vi "PrefDialog_Tabs.vi"(8 "error in (no error)":errorcluster, 11 "MyPluginsBase in":refnum<class "NHRGridSim.lvclass">) -> (0 "error out":errorcluster, 1 "Save As":bool, 2 "Changed":bool, 3 "MyPluginsBase out":refnum<class "NHRGridSim.lvclass">)   [LabVIEW 2018, in "AcPwrPlugins.lvlib" / "NHRGridSim.lvclass"]
doc: "This VI opens up the modal preference dialog window and allows a user to configure the properties with new values, or keep the existing values from the last time the function was called. The user can also save the new values to a new file name and new type name using the save as button."
uses:
  NHRGridSim.lvclass
  TypeDefs/NHRGrid_InstrumentCluster_Tabs.ctl
  TypeDefs/NHRGrid_Phases.ctl
  TypeDefs/NHRGrid_SlewRates_Tabs.ctl
  TypeDefs/NHRGrid_Configure_Tabs.ctl
  TypeDefs/NHRGrid_WaveShape_Tabs.ctl
  TypeDefs/NHRGrid_Ranges_Tabs.ctl
  TypeDefs/NHRGrid_SafetyTrips_Tabs.ctl
  Measurements.ctl
  TypeDefs/MeasurementType.ctl
  TypeDefs/NHRGrid_Modes.ctl
  TypeDefs/NHRGrid_ModeAdjust_Tabs.ctl
  <vilib>/Utility/config.llb/NI_LVConfig.lvlib
  AcPwrBaseClass/AcPwrBase.lvclass
panel:
  in  "MeasName":string
  in  "Connected":bool
  in  "ID Query":bool
  in  "Mode":T1 items=["3-Phase AC"=0, "AC"=1, "DC"=2, "AC - AC"=7, "AC - DC"=8, "DC - AC"=11, "DC - DC"=12, "2-Phase AC - AC"=5, "2-Phase AC - DC"=6, "AC - AC - AC"=3, "DC - DC - DC"=4, "AC - AC - DC"=9, "AC - DC - DC"=10, "AC - DC - AC"=13, "DC - AC - AC"=14, "DC - AC - DC"=15]
  in  "Reset":bool
  in  "Handle":string
  in  "Instruments":enum32{"Page 1", "Page 2", "Page 3"}(tab)
  in  "Instr1":T2={"Name"="", "Vout (V)"=0.0, "VType"="", "Phases"={"A-Volts (V)"=0.0, "B-Volts (V)"=0.0, "C-Volts (V)"=0.0, "Change at (Deg)"=0.0, "B-Angle (Deg)"=240.0, "C-Angle (Deg)"=120.0}, "Slew Rates"={"Vmax (V/s)"=0.0, "Vmin (V/s)"=0.0, "Imax (A/s)"=0.0, "Imin (A/s)"=0.0, "Pmax (W/s)"=0.0, "Pmin (W/s)"=0.0, "Freq Max (Hz/s)"=0.0, "Freq Min (Hz/s)"=0.0, "Ph Angle Max (Deg/s)"=0.0, "Ph Angle Min (Deg/s)"=0.0}, "FreqOut (Hz)"=60.0, "Aperture (cycles)"=1, "Configure Instrument"=0, "AC Wave Shape"=0, "Ranges"={"Voltage (V)"=0, "Current (A)"=606}, "Safety Trips"={"Vmax (V)"=0.0, "Vmin (V)"=0.0, "Vmax Time (s)"=-1.0, "Vmin Time (s)"=-1.0, "Imax Source (A)"=0.0, "Imax Sink (A)"=0.0, "I Src Time (s)"=-1.0, "I Snk Time (s)"=-1.0, "Pmax Source (W)"=0.0, "Pmax Sink (W)"=0.0, "P Src Time (s)"=-1.0, "P Snk Time (s)"=-1.0, "Abs Volt Peak"=0.0, "Enable Vpk"=FALSE, "Abs Curr Peak"=0.0, "Enable Ipk"=FALSE}} {"Safety Trips"."Abs Curr Peak" min=0.0; "Safety Trips"."Abs Volt Peak" min=0.0; "Safety Trips"."P Snk Time (s)" min=-1.0; "Safety Trips"."Pmax Sink (W)" min=0.0 format="%#_7g"; "Safety Trips"."P Src Time (s)" min=-1.0; "Safety Trips"."Pmax Source (W)" min=0.0 format="%#_7g"; "Safety Trips"."I Snk Time (s)" min=-1.0; "Safety Trips"."Imax Sink (A)" min=0.0; "Safety Trips"."I Src Time (s)" min=-1.0; "Safety Trips"."Imax Source (A)" min=0.0; "Safety Trips"."Vmax Time (s)" min=-1.0; "Safety Trips"."Vmax (V)" min=0.0; "Safety Trips"."Vmin Time (s)" min=-1.0; "Safety Trips"."Vmin (V)" min=0.0; "Ranges"."Current (A)" items=["200", "400"]; "Ranges"."Voltage (V)" items=["200", "400"]; "AC Wave Shape" items=["Sine", "User1", "User2", "User3"]; "Configure Instrument" items=["Immediate", "Sync to Phase A"]; "Aperture (cycles)" min=1 max=64; "FreqOut (Hz)" min=0.0 max=100.0; "Slew Rates"."Ph Angle Min (Deg/s)" min=0.0; "Slew Rates"."Ph Angle Max (Deg/s)" min=0.0; "Slew Rates"."Freq Min (Hz/s)" min=0.0; "Slew Rates"."Freq Max (Hz/s)" min=0.0; "Slew Rates"."Pmax (W/s)" min=0.0; "Slew Rates"."Pmin (W/s)" min=0.0; "Slew Rates"."Imax (A/s)" min=0.0; "Slew Rates"."Vmax (V/s)" min=0.0; "Slew Rates"."Imin (A/s)" min=0.0; "Slew Rates"."Vmin (V/s)" min=0.0; "Phases"."Change at (Deg)" min=0.0; "Phases"."C-Angle (Deg)" min=0.0; "Phases"."B-Angle (Deg)" min=0.0; "Phases"."C-Volts (V)" min=0.0; "Phases"."B-Volts (V)" min=0.0; "Phases"."A-Volts (V)" min=0.0; "Vout (V)" min=0.0}
  in  "Instr2":T2={"Name"="", "Vout (V)"=0.0, "VType"="", "Phases"={"A-Volts (V)"=0.0, "B-Volts (V)"=0.0, "C-Volts (V)"=0.0, "Change at (Deg)"=0.0, "B-Angle (Deg)"=240.0, "C-Angle (Deg)"=120.0}, "Slew Rates"={"Vmax (V/s)"=0.0, "Vmin (V/s)"=0.0, "Imax (A/s)"=0.0, "Imin (A/s)"=0.0, "Pmax (W/s)"=0.0, "Pmin (W/s)"=0.0, "Freq Max (Hz/s)"=0.0, "Freq Min (Hz/s)"=0.0, "Ph Angle Max (Deg/s)"=0.0, "Ph Angle Min (Deg/s)"=0.0}, "FreqOut (Hz)"=60.0, "Aperture (cycles)"=1, "Configure Instrument"=0, "AC Wave Shape"=0, "Ranges"={"Voltage (V)"=0, "Current (A)"=606}, "Safety Trips"={"Vmax (V)"=0.0, "Vmin (V)"=0.0, "Vmax Time (s)"=-1.0, "Vmin Time (s)"=-1.0, "Imax Source (A)"=0.0, "Imax Sink (A)"=0.0, "I Src Time (s)"=-1.0, "I Snk Time (s)"=-1.0, "Pmax Source (W)"=0.0, "Pmax Sink (W)"=0.0, "P Src Time (s)"=-1.0, "P Snk Time (s)"=-1.0, "Abs Volt Peak"=0.0, "Enable Vpk"=FALSE, "Abs Curr Peak"=0.0, "Enable Ipk"=FALSE}} {"Safety Trips"."Abs Curr Peak" min=0.0; "Safety Trips"."Abs Volt Peak" min=0.0; "Safety Trips"."P Snk Time (s)" min=-1.0; "Safety Trips"."Pmax Sink (W)" min=0.0 format="%#_7g"; "Safety Trips"."P Src Time (s)" min=-1.0; "Safety Trips"."Pmax Source (W)" min=0.0 format="%#_7g"; "Safety Trips"."I Snk Time (s)" min=-1.0; "Safety Trips"."Imax Sink (A)" min=0.0; "Safety Trips"."I Src Time (s)" min=-1.0; "Safety Trips"."Imax Source (A)" min=0.0; "Safety Trips"."Vmax Time (s)" min=-1.0; "Safety Trips"."Vmax (V)" min=0.0; "Safety Trips"."Vmin Time (s)" min=-1.0; "Safety Trips"."Vmin (V)" min=0.0; "Ranges"."Current (A)" items=["6", "30"]; "Ranges"."Voltage (V)" items=["175", "350"]; "AC Wave Shape" items=["Sine", "User1", "User2", "User3"]; "Configure Instrument" items=["Immediate", "Sync to Phase A"]; "Aperture (cycles)" min=1 max=64; "FreqOut (Hz)" min=0.0 max=100.0; "Slew Rates"."Ph Angle Min (Deg/s)" min=0.0; "Slew Rates"."Ph Angle Max (Deg/s)" min=0.0; "Slew Rates"."Freq Min (Hz/s)" min=0.0; "Slew Rates"."Freq Max (Hz/s)" min=0.0; "Slew Rates"."Pmax (W/s)" min=0.0; "Slew Rates"."Pmin (W/s)" min=0.0; "Slew Rates"."Imax (A/s)" min=0.0; "Slew Rates"."Vmax (V/s)" min=0.0; "Slew Rates"."Imin (A/s)" min=0.0; "Slew Rates"."Vmin (V/s)" min=0.0; "Phases"."Change at (Deg)" min=0.0; "Phases"."C-Angle (Deg)" min=0.0; "Phases"."B-Angle (Deg)" min=0.0; "Phases"."C-Volts (V)" min=0.0; "Phases"."B-Volts (V)" min=0.0; "Phases"."A-Volts (V)" min=0.0; "Vout (V)" min=0.0}
  in  "Instr3":T2={"Name"="", "Vout (V)"=0.0, "VType"="", "Phases"={"A-Volts (V)"=0.0, "B-Volts (V)"=0.0, "C-Volts (V)"=0.0, "Change at (Deg)"=0.0, "B-Angle (Deg)"=240.0, "C-Angle (Deg)"=120.0}, "Slew Rates"={"Vmax (V/s)"=0.0, "Vmin (V/s)"=0.0, "Imax (A/s)"=0.0, "Imin (A/s)"=0.0, "Pmax (W/s)"=0.0, "Pmin (W/s)"=0.0, "Freq Max (Hz/s)"=0.0, "Freq Min (Hz/s)"=0.0, "Ph Angle Max (Deg/s)"=0.0, "Ph Angle Min (Deg/s)"=0.0}, "FreqOut (Hz)"=60.0, "Aperture (cycles)"=1, "Configure Instrument"=0, "AC Wave Shape"=0, "Ranges"={"Voltage (V)"=0, "Current (A)"=606}, "Safety Trips"={"Vmax (V)"=0.0, "Vmin (V)"=0.0, "Vmax Time (s)"=-1.0, "Vmin Time (s)"=-1.0, "Imax Source (A)"=0.0, "Imax Sink (A)"=0.0, "I Src Time (s)"=-1.0, "I Snk Time (s)"=-1.0, "Pmax Source (W)"=0.0, "Pmax Sink (W)"=0.0, "P Src Time (s)"=-1.0, "P Snk Time (s)"=-1.0, "Abs Volt Peak"=0.0, "Enable Vpk"=FALSE, "Abs Curr Peak"=0.0, "Enable Ipk"=FALSE}} {"Safety Trips"."Abs Curr Peak" min=0.0; "Safety Trips"."Abs Volt Peak" min=0.0; "Safety Trips"."P Snk Time (s)" min=-1.0; "Safety Trips"."Pmax Sink (W)" min=0.0 format="%#_7g"; "Safety Trips"."P Src Time (s)" min=-1.0; "Safety Trips"."Pmax Source (W)" min=0.0 format="%#_7g"; "Safety Trips"."I Snk Time (s)" min=-1.0; "Safety Trips"."Imax Sink (A)" min=0.0; "Safety Trips"."I Src Time (s)" min=-1.0; "Safety Trips"."Imax Source (A)" min=0.0; "Safety Trips"."Vmax Time (s)" min=-1.0; "Safety Trips"."Vmax (V)" min=0.0; "Safety Trips"."Vmin Time (s)" min=-1.0; "Safety Trips"."Vmin (V)" min=0.0; "Ranges"."Current (A)" items=["6", "30"]; "Ranges"."Voltage (V)" items=["200", "400"]; "AC Wave Shape" items=["Sine", "User1", "User2", "User3"]; "Configure Instrument" items=["Immediate", "Sync to Phase A"]; "Aperture (cycles)" min=1 max=64; "FreqOut (Hz)" min=0.0 max=100.0; "Slew Rates"."Ph Angle Min (Deg/s)" min=0.0; "Slew Rates"."Ph Angle Max (Deg/s)" min=0.0; "Slew Rates"."Freq Min (Hz/s)" min=0.0; "Slew Rates"."Freq Max (Hz/s)" min=0.0; "Slew Rates"."Pmax (W/s)" min=0.0; "Slew Rates"."Pmin (W/s)" min=0.0; "Slew Rates"."Imax (A/s)" min=0.0; "Slew Rates"."Vmax (V/s)" min=0.0; "Slew Rates"."Imin (A/s)" min=0.0; "Slew Rates"."Vmin (V/s)" min=0.0; "Phases"."Change at (Deg)" min=0.0; "Phases"."C-Angle (Deg)" min=0.0; "Phases"."B-Angle (Deg)" min=0.0; "Phases"."C-Volts (V)" min=0.0; "Phases"."B-Volts (V)" min=0.0; "Phases"."A-Volts (V)" min=0.0; "Vout (V)" min=0.0}
  in  "Measurements":T9 {"Instrument Number" items=["1", "2", "3"]}
  in  "btnSaveAs":bool
  in  "Measurement RefreshTime (ms)":u32
  in  "btnSave":bool
  in  "btnCancel":bool
  # "Voltages (L-N)"
  # "Voltages (L-N)"
  # "Voltages (L-N)"
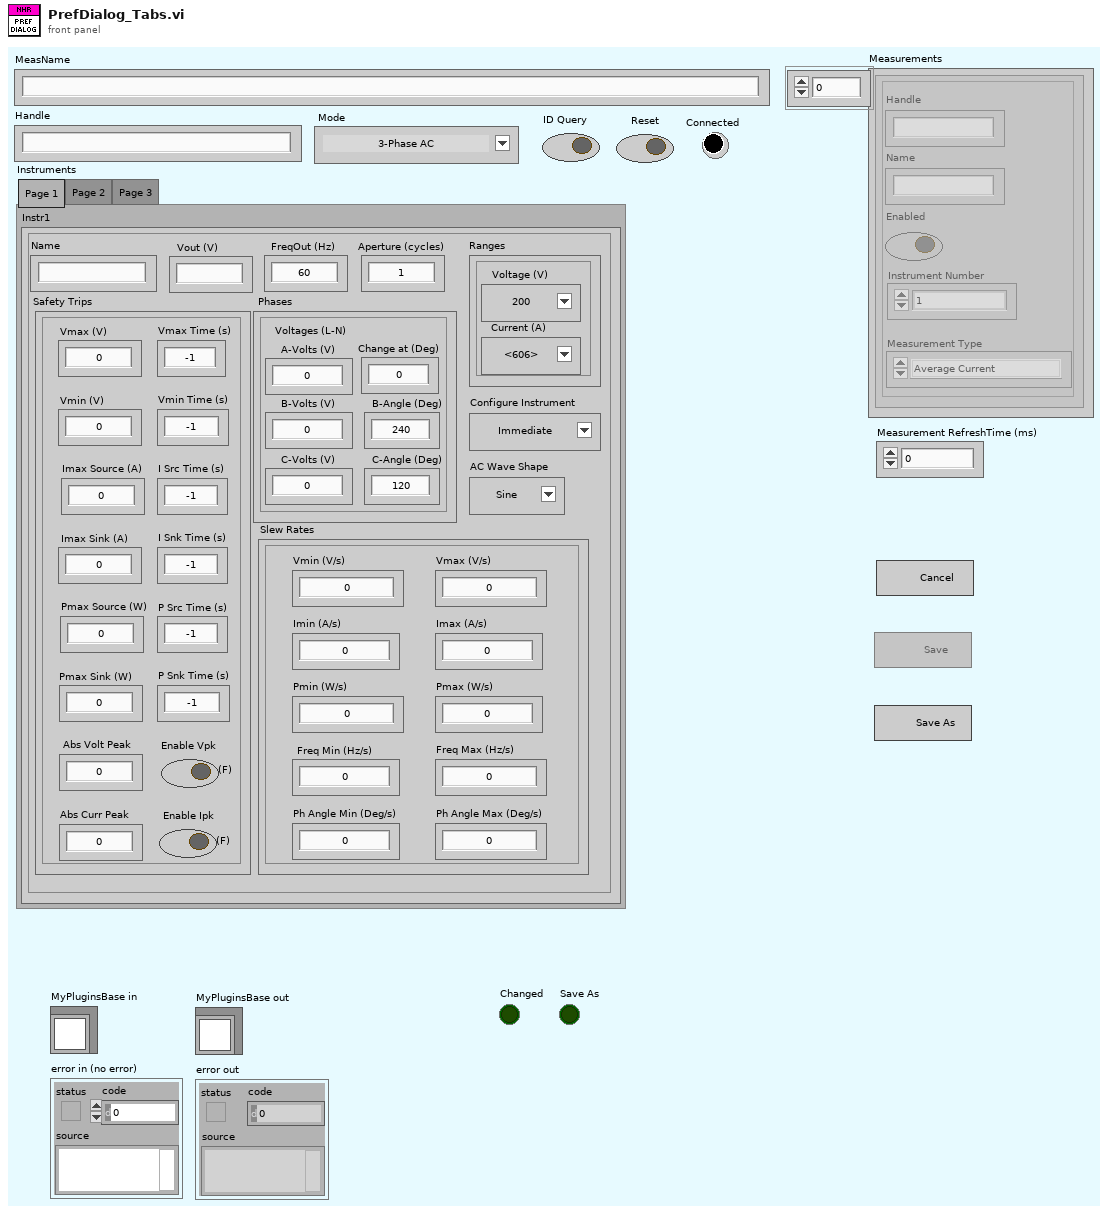
[diagram p1: front panel]
types:
  T1 = typedef "AcPwrPlugins.lvlib/NHRGridSim.lvclass/NHRGrid_Modes.ctl" = u8
  T2 = typedef "AcPwrPlugins.lvlib/NHRGridSim.lvclass/NHRGrid_InstrumentCluster_Tabs.ctl" = cluster{"Name":string, "Vout (V)":dbl, "VType":string, "Phases":T3, "Slew Rates":T4, "FreqOut (Hz)":dbl, "Aperture (cycles)":i32, "Configure Instrument":T5, "AC Wave Shape":T6, "Ranges":T7, "Safety Trips":T8}
  T3 = typedef "AcPwrPlugins.lvlib/NHRGridSim.lvclass/NHRGrid_Phases.ctl" = cluster{"A-Volts (V)":dbl, "B-Volts (V)":dbl, "C-Volts (V)":dbl, "Change at (Deg)":dbl, "B-Angle (Deg)":dbl, "C-Angle (Deg)":dbl}
  T4 = typedef "AcPwrPlugins.lvlib/NHRGridSim.lvclass/NHRGrid_SlewRates_Tabs.ctl" = cluster{"Vmax (V/s)":dbl, "Vmin (V/s)":dbl, "Imax (A/s)":dbl, "Imin (A/s)":dbl, "Pmax (W/s)":dbl, "Pmin (W/s)":dbl, "Freq Max (Hz/s)":dbl, "Freq Min (Hz/s)":dbl, "Ph Angle Max (Deg/s)":dbl, "Ph Angle Min (Deg/s)":dbl}
  T5 = typedef "AcPwrPlugins.lvlib/NHRGridSim.lvclass/NHRGrid_Configure_Tabs.ctl" = u16
  T6 = typedef "AcPwrPlugins.lvlib/NHRGridSim.lvclass/NHRGrid_WaveShape_Tabs.ctl" = u16
  T7 = typedef "AcPwrPlugins.lvlib/NHRGridSim.lvclass/NHRGrid_Ranges_Tabs.ctl" = cluster{"Voltage (V)":u16, "Current (A)":u16}
  T8 = typedef "AcPwrPlugins.lvlib/NHRGridSim.lvclass/NHRGrid_SafetyTrips_Tabs.ctl" = cluster{"Vmax (V)":dbl, "Vmin (V)":dbl, "Vmax Time (s)":dbl, "Vmin Time (s)":dbl, "Imax Source (A)":dbl, "Imax Sink (A)":dbl, "I Src Time (s)":dbl, "I Snk Time (s)":dbl, "Pmax Source (W)":dbl, "Pmax Sink (W)":dbl, "P Src Time (s)":dbl, "P Snk Time (s)":dbl, "Abs Volt Peak":dbl, "Enable Vpk":bool, "Abs Curr Peak":dbl, "Enable Ipk":bool}
  T9 = typedef "AcPwrPlugins.lvlib/NHRGridSim.lvclass/Measurements.ctl" = cluster{"Handle":string, "Name":string, "Enabled ":bool, "Measurement Value":dbl, "Instrument Number ":i32, "Measurement Type ":T10}[]
  T10 = typedef "AcPwrPlugins.lvlib/NHRGridSim.lvclass/MeasurementType.ctl" = enum16{"Average Current", "Average Voltage"}
  T11 = enum32{"Invalid", "Default", "Floating", "Floating/Auto-Hide", "Modal"}
  T12 = enum32{"Invalid", "Standard", "Closed", "Hidden", "Minimized", "Maximized"}
  T13 = typedef "AcPwrPlugins.lvlib/NHRGridSim.lvclass/NHRGrid_ModeAdjust_Tabs.ctl" = enum16{"ShowTabs", "InstrNames", "VoltRanges", "ConfigOpts"}
  T14 = enum8{"Enabled", "Disabled", "Disabled and Grayed Out"}
  T15 = typedef "AcPwrPlugins.lvlib/AcPwrBase.lvclass/BaseConfig.ctl" = cluster{"Frequency":dbl, "FrequencyRange":dbl[], "Phases":T16[], "Name":string, "PluginConfigVariant":variant, "PluginMeasVariant":variant}
  T16 = typedef "AcPwrPlugins.lvlib/AcPwrBase.lvclass/Phase.ctl" = cluster{"Name":string, "Enabled":bool, "VoltageLevel":dbl, "Handle":string, "VoltageRange":dbl[], "Connected":bool, "CurrentLimit":dbl, "Waveform":string}
  T17 = typedef "AcPwrPlugins.lvlib/AcPwrBase.lvclass/BaseMeasurements.ctl" = cluster{"Handle":string, "Name":string, "Enabled":bool, "Measurement Value":dbl, "btnMeasFetch":bool, "Chroma Hold Peak Current Measurement":bool, "Chroma Measurement Type":T18, "Chroma Protection Status String":string, "NHRDC Fetch Method":i32, "NHRDC Fetch Time (s)":sgl, "NHRDC Measurement Type":i32, "NHRGridSim Measurement Type ":enum16{"Average Current", "Max Current", "Min Current", "Average Voltage", "Max Voltage", "Min Voltage", "Average True Power", "Max True Power", "Min True Power", "Average Apparent Power", "Max Apparent Power", "Min Apparent Power", "Power Factor", "Crest Factor"}, "NHRGridSim Phase ":i32, "PPS Measurement Type ":enum16{"Voltage RMS L-N", "Voltage RMS L-L", "Frequency", "Current RMS", "Current Peak", "Crest Factor", "Power Factor", "Power VA", "Real Power"}, "PPS Channel Name":enum16{"A", "B", "C"}}[]
  T18 = typedef "AcPwrPlugins.lvlib/ChromaAcLoad.lvclass/MeasurementType.ctl" = enum16{"Voltage (Vrms or V)", "Current (Arms or A)", "Power (W)", "Peak Voltage (V)", "Peak Current (A)", "Peak Power (W)", "Frequency (Hz)", "Resistance (Ohms)", "Voltage Overshoot (V)", "Positive Peak Current (A)", "Voltage Undershoot (V)", "Negative Peak Current (A)", "Apparent Power (VA)", "Reacitive Power (VAR)", "Voltage THD", "Power Factor", "Current's Crest Factor"}
  T19 = typedef "NI_LVConfig.lvlib/Config Data RefNum.ctl" = refnum<k1>
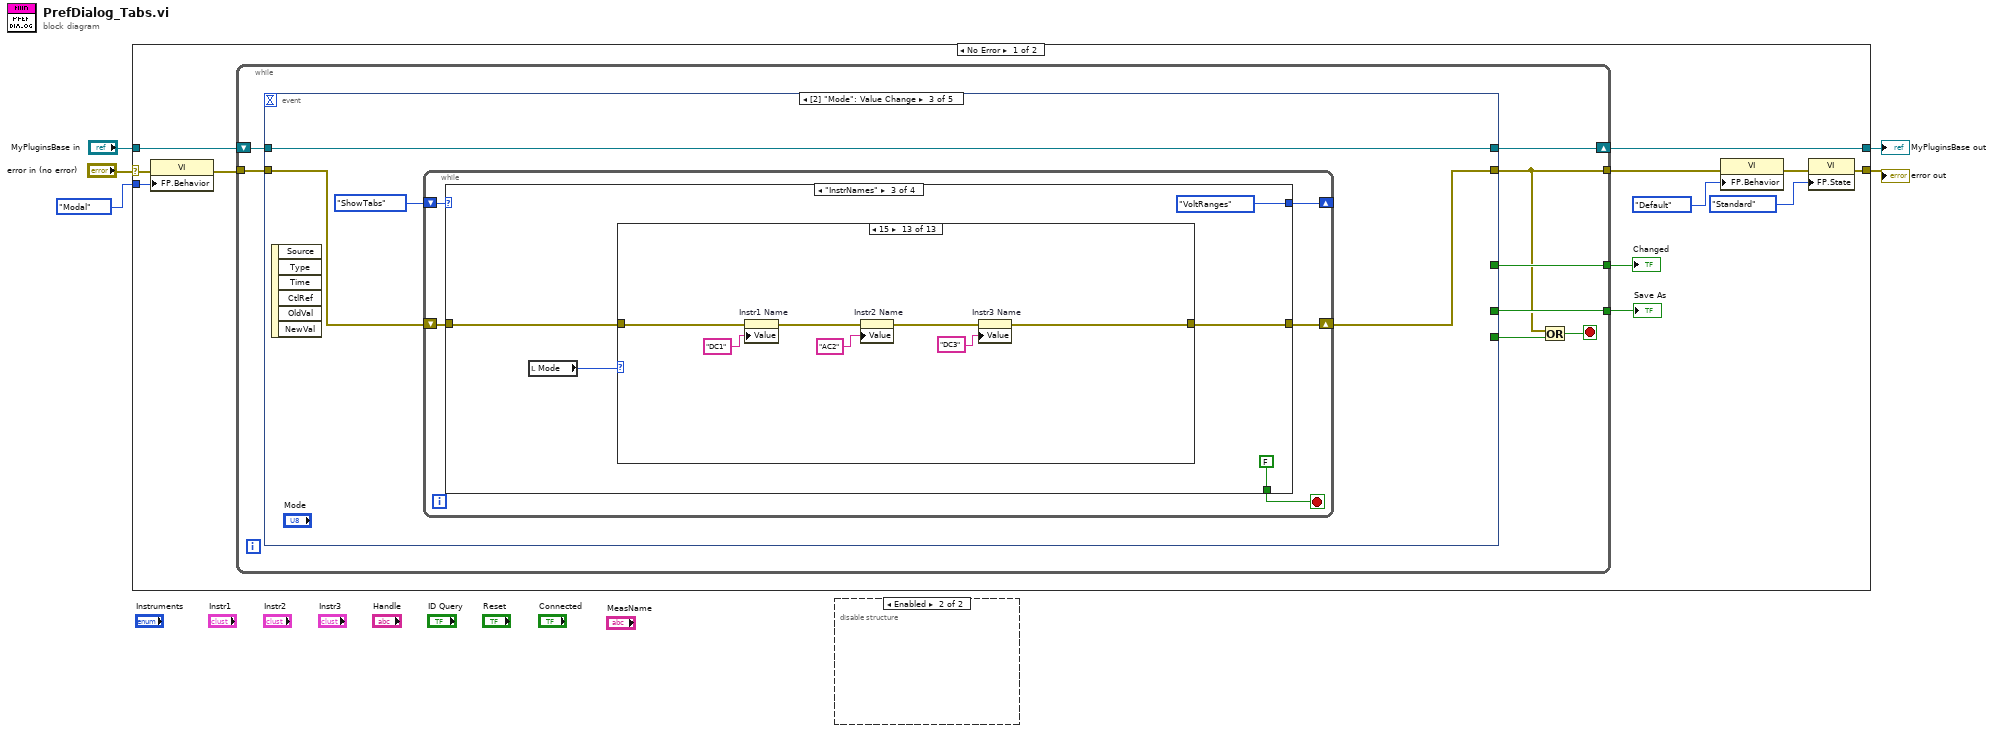
[diagram p0: block diagram]
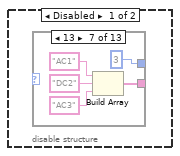
[diagram p2: hidden frame]
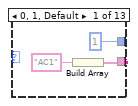
[diagram p3: hidden frame]
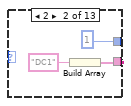
[diagram p4: hidden frame]
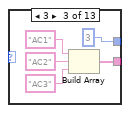
[diagram p5: hidden frame]
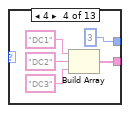
[diagram p6: hidden frame]
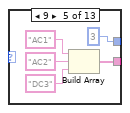
[diagram p7: hidden frame]
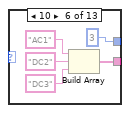
[diagram p8: hidden frame]
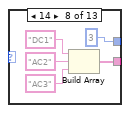
[diagram p9: hidden frame]
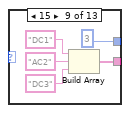
[diagram p10: hidden frame]
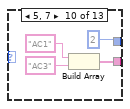
[diagram p11: hidden frame]
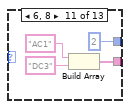
[diagram p12: hidden frame]
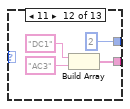
[diagram p13: hidden frame]
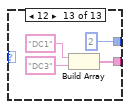
[diagram p14: hidden frame]
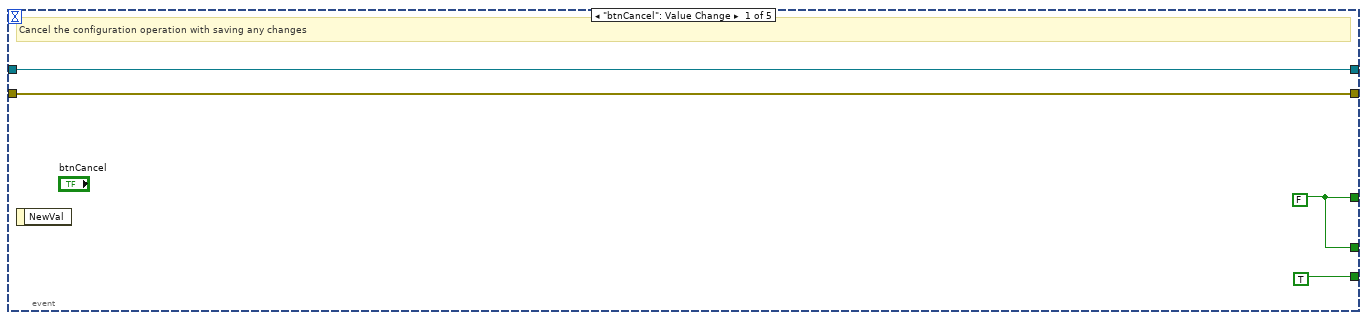
[diagram p15: hidden frame]
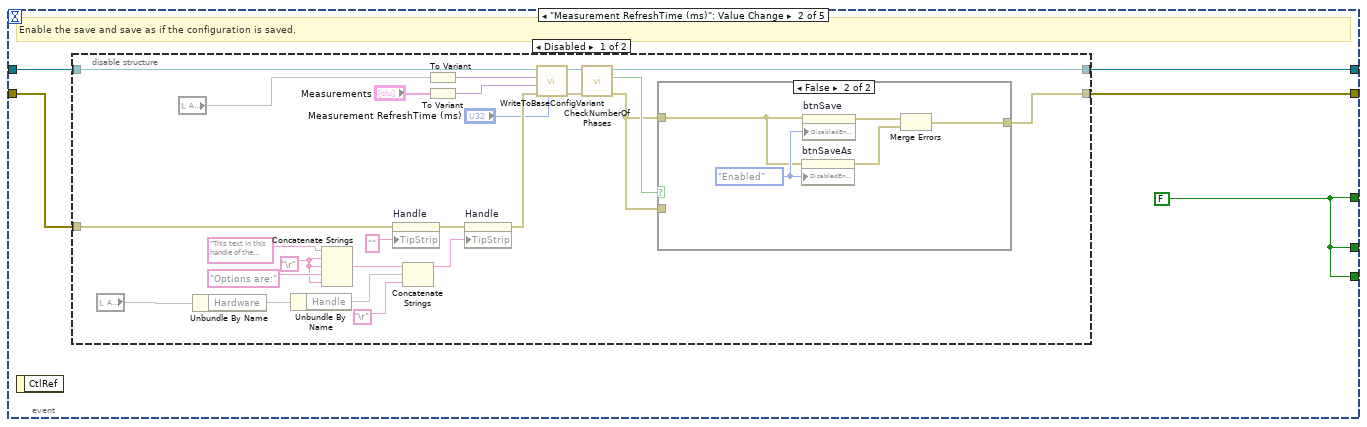
[diagram p16: hidden frame]
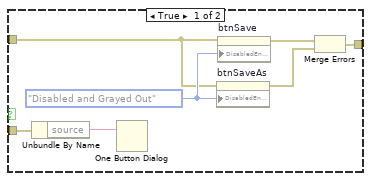
[diagram p17: hidden frame]
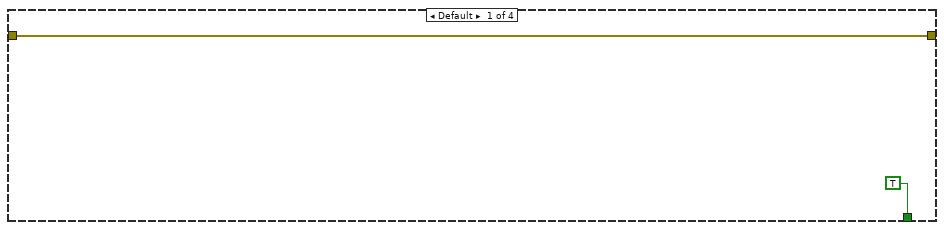
[diagram p19: hidden frame]
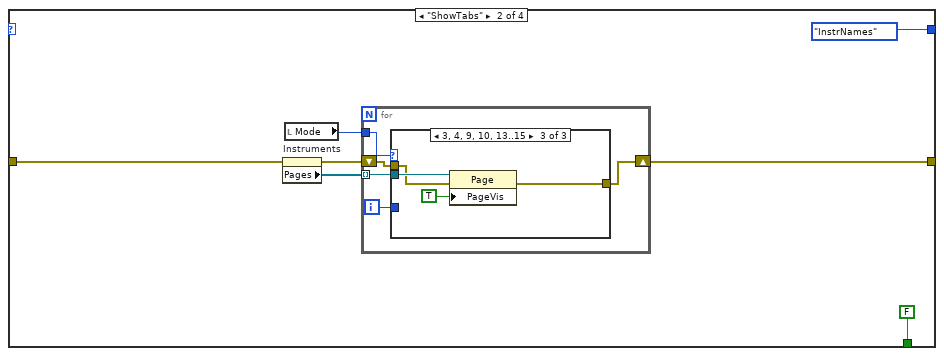
[diagram p20: hidden frame]
diagram:
  n1 = case shown="No Error" "error in (no error)" {
    selector: "error in (no error)" -> [w16 w476]
    tunnel: "MyPluginsBase in" -> [w7 w475]
    tunnel: [w12 w475] -> w3
    tunnel: [w10 w476] -> w2
    tunnel: T11."Modal" ("Front Panel Window:Behavior") -> [w8 _]
    frame No Error {
      n2 = property class="VI"(error in=w16, "FP.Behavior"=w8) -> (error out=w6:errorcluster)  [unwired: 1 in, 1 out]
      n3 = while {
        shift-right: [w23] -> w12
        shift-left: w7 -> [w24]
        tunnel: [w25] -> w17
        tunnel: [w21] -> w11
        tunnel: w6 -> [w22]
        tunnel: [w18] -> w9
        stop <- w20 stop-if-true
        n4 = event shown="[2] \"Mode\": Value Change" {
          selector: _ -> [_ _ _ _ _]
          dyn-events: _ -> [_ _ _ _ _]
          timeout: _ -> [_ _ _ _ _]
          tunnel: [w26 w33 _ w390 w427] -> w25
          tunnel: [TRUE w33 _ w390 w427] -> w19
          tunnel: w24 -> [w28 w31 w77 w387 w426]
          tunnel: [w28 w32 w77 w388 w423] -> w23
          tunnel: [w27 w34 w74 w389 w424] -> w18
          tunnel: w22 -> [w27 w30 w75 w386 w425]
          tunnel: [w26 w33 _ FALSE w427] -> w21
          event "btnCancel": Value Change {
            w26 = FALSE
            # "Cancel the configuration operation with saving any changes"
            n5 = event-data() -> ()  [unwired: 1 in, 1 out]
          }
          event "Measurement RefreshTime (ms)": Value Change {
            w33 = FALSE
            # "Enable the save and save as if the configuration is saved."
            n6 = event-data() -> ()  [unwired: 1 in, 1 out]
            n7 = disable-structure shown="Disabled" {
              disable-tunnel: [w59 w72] -> w34
              disable-tunnel: [w54 w73] -> w32
              disable-tunnel: w31 -> [w51 w73]
              disable-tunnel: w30 -> [w45 w72]
              frame Disabled {
                w56 = "\r"
                n8 = local read item#-1() -> (w35)
                n9 = local read item#-1() -> (w36)
                n10 = Unbundle By Name(w35) -> ("Hardware"=w47)
                n11 = Unbundle By Name(w47) -> ("Handle"=w38)
                n12 = Concatenate Strings("This text in this handle of the instrument and entered in the  \nhandle control in the Phases array EXACTLY, lest the attempt \nto interact with the instrument will fail.", w56, w56, "Options are:" ("Handle"), w56) -> (w55:string)
                n13 = property on="Handle" class="Str"(error in=w45, "TipStrip"="" ("Tip Strip")) -> (error out=w43:errorcluster)  [unwired: 1 in, 1 out]
                n14 = Concatenate Strings(w55, w38, "\r") -> (w42:string)
                n15 = To Variant(anything=w36) -> (Variant=w52:variant)
                n16 = To Variant(anything="Measurements") -> (Variant=w39:variant)
                n17 = property on="Handle" class="Str"(error in=w43, "TipStrip"=w42) -> (error out=w44:errorcluster)  [unwired: 1 in, 1 out]
                n18 = call "WriteToBaseConfigVariant.vi"("Measurement RefreshTime (ms)"="Measurement RefreshTime (ms)", "error in (no error)"=w44, "Meas"=w39, "Config"=w52, "NHRGridSim in"=w51) -> ("error out"=w49:errorcluster, "NHRGridSim out"=w50:refnum<class "NHRGridSim.lvclass">)  [unwired: 5 in]
                n19 = call "CheckNumberOfPhases.vi"("error in (no error)"=w49, "NHRGridSim in"=w50) -> ("error out"=w48:errorcluster, "Boolean"=w53:bool, "NHRGridSim out"=w54:refnum<class "NHRGridSim.lvclass">)  [unwired: 6 in, 1 out]
                n20 = case shown="False" w53 {
                  tunnel: w48 -> [w63 w68]
                  tunnel: [w62 w67] -> w59
                  tunnel: w48 -> [w60 _]
                  frame True {
                    w64 = T14."Disabled and Grayed Out" ("Disabled")
                    n21 = Unbundle By Name(w60) -> ("source"=w61:string)
                    n22 = One Button Dialog(message=w61) -> ()  [unwired: 1 in, 1 out]
                    n23 = property on="btnSaveAs" class="Bool"(error in=w63, "DisabledEnum"=w64) -> (error out=w66:errorcluster)  [unwired: 1 in, 1 out]
                    n24 = property on="btnSave" class="Bool"(error in=w63, "DisabledEnum"=w64) -> (error out=w65:errorcluster)  [unwired: 1 in, 1 out]
                    n25 = Merge Errors(w65, w66) -> (w62:errorcluster)
                  }
                  frame False {
                    w69 = T14."Enabled" ("Disabled")
                    n26 = property on="btnSaveAs" class="Bool"(error in=w68, "DisabledEnum"=w69) -> (error out=w71:errorcluster)  [unwired: 1 in, 1 out]
                    n27 = property on="btnSave" class="Bool"(error in=w68, "DisabledEnum"=w69) -> (error out=w70:errorcluster)  [unwired: 1 in, 1 out]
                    n28 = Merge Errors(w70, w71) -> (w67:errorcluster)
                  }
                }
              }
              frame Enabled {
              }
            }
          }
          event Value Change {
            n29 = event-data() -> ()  [unwired: 1 in, 6 out]
            n30 = while {
              shift-right: [w79] -> _
              shift-left: NHRGrid_ModeAdjust_Tabs."ShowTabs" ("AcPwrPlugins.lvlib:NHRGridSim.lvclass:NHRGrid_ModeAdjust_Tabs") -> [w82]
              shift-right: [w80] -> w74
              shift-left: w75 -> [w81]
              stop <- w78 stop-if-true
              n31 = case shown="\"InstrNames\"" w82 {
                tunnel: w81 -> [w83 w89 w120 w216]
                tunnel: [w83 w87 w119 w215] -> w80
                tunnel: [_ NHRGrid_ModeAdjust_Tabs."InstrNames" ("AcPwrPlugins.lvlib:NHRGridSim.lvclass:NHRGrid_ModeAdjust_Tabs") NHRGrid_ModeAdjust_Tabs."VoltRanges" ("AcPwrPlugins.lvlib:NHRGridSim.lvclass:NHRGrid_ModeAdjust_Tabs") NHRGrid_ModeAdjust_Tabs."ConfigOpts" ("AcPwrPlugins.lvlib:NHRGridSim.lvclass:NHRGrid_ModeAdjust_Tabs")] -> w79
                tunnel: [TRUE FALSE FALSE FALSE] -> w78
                frame Default {
                }
                frame "ShowTabs" {
                  n32 = property on="Instruments" class="TabCtl (strict)"(error in=w89) -> (error out=w88:errorcluster, "Pages"=w91:refnum<vi>[])  [unwired: 1 in, 1 out]
                  n33 = local read "Mode"() -> (w90:T1)
                  n34 = for {
                    tunnel: w91 -> [w95] mode=indexing
                    tunnel: w90 -> [w96]
                    shift-right: [w92] -> w87
                    shift-left: w88 -> [w93]
                    i -> [w94]
                    n35 = case shown="3, 4, 9, 10, 13..15" w96 {
                      tunnel: w95 -> [w105 w114 w118]
                      tunnel: w94 -> [w100 w109 _]
                      tunnel: w93 -> [w98 w107 w116]
                      tunnel: [w97 w106 w115] -> w92
                      frame 0..2, Default {
                        n36 = Equal?(x=0, y=w100) -> (x = y?=w101:bool)
                        n37 = Select(t=TRUE ("x .or. y?"), s=w101, f=FALSE ("x .or. y?")) -> (s? t:f=w104:bool)
                        n38 = property class="Page"(reference=w105, error in=w98, "PageVis"=w104) -> (error out=w97:errorcluster)  [unwired: 1 out]
                      }
                      frame 5..8, 11, 12 {
                        n39 = Equal?(x=1, y=w109) -> (x = y?=w110:bool)
                        n40 = Select(t=FALSE ("x .or. y?"), s=w110, f=TRUE ("x .or. y?")) -> (s? t:f=w113:bool)
                        n41 = property class="Page"(reference=w114, error in=w107, "PageVis"=w113) -> (error out=w106:errorcluster)  [unwired: 1 out]
                      }
                      frame 3, 4, 9, 10, 13..15 {
                        n42 = property class="Page"(reference=w118, error in=w116, "PageVis"=TRUE ("x .or. y?")) -> (error out=w115:errorcluster)  [unwired: 1 out]
                      }
                    }
                  }
                }
                frame "InstrNames" {
                  n43 = local read "Mode"() -> (w121:T1)
                  n44 = case shown="15" w121 {
                    tunnel: w120 -> [w129 w136 w143 w150 w157 w164 w171 w178 w185 w192 w199 w206 w213]
                    tunnel: [w126 w133 w140 w147 w154 w161 w168 w175 w182 w189 w196 w203 w210] -> w119
                    frame 0, 1, Default {
                      n45 = property on="Instr1 Name" class="Str"(error in=w129, "Value"="AC1") -> (error out=w128:errorcluster)  [unwired: 1 in, 1 out]
                      n46 = property on="Instr2 Name" class="Str"(error in=w128, "Value"="N/A") -> (error out=w127:errorcluster)  [unwired: 1 in, 1 out]
                      n47 = property on="Instr3 Name" class="Str"(error in=w127, "Value"="N/A") -> (error out=w126:errorcluster)  [unwired: 1 in, 1 out]
                    }
                    frame 2 {
                      n48 = property on="Instr1 Name" class="Str"(error in=w136, "Value"="DC1") -> (error out=w135:errorcluster)  [unwired: 1 in, 1 out]
                      n49 = property on="Instr2 Name" class="Str"(error in=w135, "Value"="N/A") -> (error out=w134:errorcluster)  [unwired: 1 in, 1 out]
                      n50 = property on="Instr3 Name" class="Str"(error in=w134, "Value"="N/A") -> (error out=w133:errorcluster)  [unwired: 1 in, 1 out]
                    }
                    frame 5, 7 {
                      n51 = property on="Instr1 Name" class="Str"(error in=w143, "Value"="AC1") -> (error out=w142:errorcluster)  [unwired: 1 in, 1 out]
                      n52 = property on="Instr2 Name" class="Str"(error in=w142, "Value"="N/A") -> (error out=w141:errorcluster)  [unwired: 1 in, 1 out]
                      n53 = property on="Instr3 Name" class="Str"(error in=w141, "Value"="AC3") -> (error out=w140:errorcluster)  [unwired: 1 in, 1 out]
                    }
                    frame 6, 8 {
                      n54 = property on="Instr1 Name" class="Str"(error in=w150, "Value"="AC1") -> (error out=w149:errorcluster)  [unwired: 1 in, 1 out]
                      n55 = property on="Instr2 Name" class="Str"(error in=w149, "Value"="N/A") -> (error out=w148:errorcluster)  [unwired: 1 in, 1 out]
                      n56 = property on="Instr3 Name" class="Str"(error in=w148, "Value"="DC3") -> (error out=w147:errorcluster)  [unwired: 1 in, 1 out]
                    }
                    frame 11 {
                      n57 = property on="Instr1 Name" class="Str"(error in=w157, "Value"="DC1") -> (error out=w156:errorcluster)  [unwired: 1 in, 1 out]
                      n58 = property on="Instr2 Name" class="Str"(error in=w156, "Value"="N/A") -> (error out=w155:errorcluster)  [unwired: 1 in, 1 out]
                      n59 = property on="Instr3 Name" class="Str"(error in=w155, "Value"="AC3") -> (error out=w154:errorcluster)  [unwired: 1 in, 1 out]
                    }
                    frame 12 {
                      n60 = property on="Instr1 Name" class="Str"(error in=w164, "Value"="DC1") -> (error out=w163:errorcluster)  [unwired: 1 in, 1 out]
                      n61 = property on="Instr2 Name" class="Str"(error in=w163, "Value"="N/A") -> (error out=w162:errorcluster)  [unwired: 1 in, 1 out]
                      n62 = property on="Instr3 Name" class="Str"(error in=w162, "Value"="DC3") -> (error out=w161:errorcluster)  [unwired: 1 in, 1 out]
                    }
                    frame 3 {
                      n63 = property on="Instr1 Name" class="Str"(error in=w171, "Value"="AC1") -> (error out=w170:errorcluster)  [unwired: 1 in, 1 out]
                      n64 = property on="Instr2 Name" class="Str"(error in=w170, "Value"="AC2") -> (error out=w169:errorcluster)  [unwired: 1 in, 1 out]
                      n65 = property on="Instr3 Name" class="Str"(error in=w169, "Value"="AC3") -> (error out=w168:errorcluster)  [unwired: 1 in, 1 out]
                    }
                    frame 4 {
                      n66 = property on="Instr1 Name" class="Str"(error in=w178, "Value"="DC1") -> (error out=w177:errorcluster)  [unwired: 1 in, 1 out]
                      n67 = property on="Instr2 Name" class="Str"(error in=w177, "Value"="DC2") -> (error out=w176:errorcluster)  [unwired: 1 in, 1 out]
                      n68 = property on="Instr3 Name" class="Str"(error in=w176, "Value"="DC3") -> (error out=w175:errorcluster)  [unwired: 1 in, 1 out]
                    }
                    frame 9 {
                      n69 = property on="Instr1 Name" class="Str"(error in=w185, "Value"="AC1") -> (error out=w184:errorcluster)  [unwired: 1 in, 1 out]
                      n70 = property on="Instr2 Name" class="Str"(error in=w184, "Value"="AC2") -> (error out=w183:errorcluster)  [unwired: 1 in, 1 out]
                      n71 = property on="Instr3 Name" class="Str"(error in=w183, "Value"="DC3") -> (error out=w182:errorcluster)  [unwired: 1 in, 1 out]
                    }
                    frame 10 {
                      n72 = property on="Instr1 Name" class="Str"(error in=w192, "Value"="AC1") -> (error out=w191:errorcluster)  [unwired: 1 in, 1 out]
                      n73 = property on="Instr2 Name" class="Str"(error in=w191, "Value"="DC2") -> (error out=w190:errorcluster)  [unwired: 1 in, 1 out]
                      n74 = property on="Instr3 Name" class="Str"(error in=w190, "Value"="DC3") -> (error out=w189:errorcluster)  [unwired: 1 in, 1 out]
                    }
                    frame 13 {
                      n75 = property on="Instr1 Name" class="Str"(error in=w199, "Value"="AC1") -> (error out=w198:errorcluster)  [unwired: 1 in, 1 out]
                      n76 = property on="Instr2 Name" class="Str"(error in=w198, "Value"="DC2") -> (error out=w197:errorcluster)  [unwired: 1 in, 1 out]
                      n77 = property on="Instr3 Name" class="Str"(error in=w197, "Value"="AC3") -> (error out=w196:errorcluster)  [unwired: 1 in, 1 out]
                    }
                    frame 14 {
                      n78 = property on="Instr1 Name" class="Str"(error in=w206, "Value"="DC1") -> (error out=w205:errorcluster)  [unwired: 1 in, 1 out]
                      n79 = property on="Instr2 Name" class="Str"(error in=w205, "Value"="AC2") -> (error out=w204:errorcluster)  [unwired: 1 in, 1 out]
                      n80 = property on="Instr3 Name" class="Str"(error in=w204, "Value"="AC3") -> (error out=w203:errorcluster)  [unwired: 1 in, 1 out]
                    }
                    frame 15 {
                      n81 = property on="Instr1 Name" class="Str"(error in=w213, "Value"="DC1") -> (error out=w212:errorcluster)  [unwired: 1 in, 1 out]
                      n82 = property on="Instr2 Name" class="Str"(error in=w212, "Value"="AC2") -> (error out=w211:errorcluster)  [unwired: 1 in, 1 out]
                      n83 = property on="Instr3 Name" class="Str"(error in=w211, "Value"="DC3") -> (error out=w210:errorcluster)  [unwired: 1 in, 1 out]
                    }
                  }
                }
                frame "VoltRanges" {
                  n84 = local read "Mode"() -> (w217:T1)
                  n85 = case shown="15" w217 {
                    tunnel: w216 -> [w226 w236 w249 w262 w273 w283 w293 w303 w315 w328 w338 w348 w358 w366 w376 w383]
                    tunnel: [w223 w233 w246 w259 w270 w280 w290 w300 w312 w325 w335 w345 w355 w363 w373 w380] -> w215
                    frame 0, Default {
                      n86 = Build Array("303" ("element"), "606" ("element")) -> (w227:string[])
                      n87 = property on="Instr1 Voltage (V)" class="Ring (strict)"(error in=w226, "Strings []"=w227) -> (error out=w225:errorcluster)  [unwired: 1 in, 1 out]
                      n88 = Build Array("0" ("element"), "0" ("element")) -> (w220:string[])
                      n89 = property on="Instr2 Voltage (V)" class="Ring (strict)"(error in=w225, "Strings []"=w220) -> (error out=w224:errorcluster)  [unwired: 1 in, 1 out]
                      n90 = property on="Instr3 Voltage (V)" class="Ring (strict)"(error in=w224, "Strings []"=w220) -> (error out=w223:errorcluster)  [unwired: 1 in, 1 out]
                    }
                    frame 10 {
                      n91 = Build Array("175" ("element"), "350" ("element")) -> (w237:string[])
                      n92 = property on="Instr1 Voltage (V)" class="Ring (strict)"(error in=w236, "Strings []"=w237) -> (error out=w235:errorcluster)  [unwired: 1 in, 1 out]
                      n93 = Build Array("200" ("element"), "400" ("element")) -> (w230:string[])
                      n94 = property on="Instr2 Voltage (V)" class="Ring (strict)"(error in=w235, "Strings []"=w230) -> (error out=w234:errorcluster)  [unwired: 1 in, 1 out]
                      n95 = property on="Instr3 Voltage (V)" class="Ring (strict)"(error in=w234, "Strings []"=w230) -> (error out=w233:errorcluster)  [unwired: 1 in, 1 out]
                    }
                    frame 5 {
                      n96 = Build Array("350" ("element"), "500" ("element")) -> (w250:string[])
                      n97 = property on="Instr1 Voltage (V)" class="Ring (strict)"(error in=w249, "Strings []"=w250) -> (error out=w248:errorcluster)  [unwired: 1 in, 1 out]
                      n98 = Build Array("0" ("element"), "0" ("element")) -> (w243:string[])
                      n99 = property on="Instr2 Voltage (V)" class="Ring (strict)"(error in=w248, "Strings []"=w243) -> (error out=w247:errorcluster)  [unwired: 1 in, 1 out]
                      n100 = Build Array("175" ("element"), "350" ("element")) -> (w240:string[])
                      n101 = property on="Instr3 Voltage (V)" class="Ring (strict)"(error in=w247, "Strings []"=w240) -> (error out=w246:errorcluster)  [unwired: 1 in, 1 out]
                    }
                    frame 11 {
                      n102 = Build Array("200" ("element"), "400" ("element")) -> (w263:string[])
                      n103 = property on="Instr1 Voltage (V)" class="Ring (strict)"(error in=w262, "Strings []"=w263) -> (error out=w261:errorcluster)  [unwired: 1 in, 1 out]
                      n104 = Build Array("0" ("element"), "0" ("element")) -> (w256:string[])
                      n105 = property on="Instr2 Voltage (V)" class="Ring (strict)"(error in=w261, "Strings []"=w256) -> (error out=w260:errorcluster)  [unwired: 1 in, 1 out]
                      n106 = Build Array("175" ("element"), "350" ("element")) -> (w253:string[])
                      n107 = property on="Instr3 Voltage (V)" class="Ring (strict)"(error in=w260, "Strings []"=w253) -> (error out=w259:errorcluster)  [unwired: 1 in, 1 out]
                    }
                    frame 12 {
                      n108 = Build Array("200" ("element"), "400" ("element")) -> (w266:string[])
                      n109 = property on="Instr1 Voltage (V)" class="Ring (strict)"(error in=w273, "Strings []"=w266) -> (error out=w272:errorcluster)  [unwired: 1 in, 1 out]
                      n110 = Build Array("0" ("element"), "0" ("element")) -> (w267:string[])
                      n111 = property on="Instr2 Voltage (V)" class="Ring (strict)"(error in=w272, "Strings []"=w267) -> (error out=w271:errorcluster)  [unwired: 1 in, 1 out]
                      n112 = property on="Instr3 Voltage (V)" class="Ring (strict)"(error in=w271, "Strings []"=w266) -> (error out=w270:errorcluster)  [unwired: 1 in, 1 out]
                    }
                    frame 15 {
                      n113 = Build Array("200" ("element"), "400" ("element")) -> (w276:string[])
                      n114 = property on="Instr1 Voltage (V)" class="Ring (strict)"(error in=w283, "Strings []"=w276) -> (error out=w282:errorcluster)  [unwired: 1 in, 1 out]
                      n115 = Build Array("175" ("element"), "350" ("element")) -> (w277:string[])
                      n116 = property on="Instr2 Voltage (V)" class="Ring (strict)"(error in=w282, "Strings []"=w277) -> (error out=w281:errorcluster)  [unwired: 1 in, 1 out]
                      n117 = property on="Instr3 Voltage (V)" class="Ring (strict)"(error in=w281, "Strings []"=w276) -> (error out=w280:errorcluster)  [unwired: 1 in, 1 out]
                    }
                    frame 13 {
                      n118 = Build Array("175" ("element"), "350" ("element")) -> (w286:string[])
                      n119 = property on="Instr1 Voltage (V)" class="Ring (strict)"(error in=w293, "Strings []"=w286) -> (error out=w292:errorcluster)  [unwired: 1 in, 1 out]
                      n120 = Build Array("200" ("element"), "400" ("element")) -> (w287:string[])
                      n121 = property on="Instr2 Voltage (V)" class="Ring (strict)"(error in=w292, "Strings []"=w287) -> (error out=w291:errorcluster)  [unwired: 1 in, 1 out]
                      n122 = property on="Instr3 Voltage (V)" class="Ring (strict)"(error in=w291, "Strings []"=w286) -> (error out=w290:errorcluster)  [unwired: 1 in, 1 out]
                    }
                    frame 7 {
                      n123 = Build Array("175" ("element"), "350" ("element")) -> (w296:string[])
                      n124 = property on="Instr1 Voltage (V)" class="Ring (strict)"(error in=w303, "Strings []"=w296) -> (error out=w302:errorcluster)  [unwired: 1 in, 1 out]
                      n125 = Build Array("0" ("element"), "0" ("element")) -> (w297:string[])
                      n126 = property on="Instr2 Voltage (V)" class="Ring (strict)"(error in=w302, "Strings []"=w297) -> (error out=w301:errorcluster)  [unwired: 1 in, 1 out]
                      n127 = property on="Instr3 Voltage (V)" class="Ring (strict)"(error in=w301, "Strings []"=w296) -> (error out=w300:errorcluster)  [unwired: 1 in, 1 out]
                    }
                    frame 6 {
                      n128 = Build Array("350" ("element"), "500" ("element")) -> (w316:string[])
                      n129 = property on="Instr1 Voltage (V)" class="Ring (strict)"(error in=w315, "Strings []"=w316) -> (error out=w314:errorcluster)  [unwired: 1 in, 1 out]
                      n130 = Build Array("0" ("element"), "0" ("element")) -> (w309:string[])
                      n131 = property on="Instr2 Voltage (V)" class="Ring (strict)"(error in=w314, "Strings []"=w309) -> (error out=w313:errorcluster)  [unwired: 1 in, 1 out]
                      n132 = Build Array("200" ("element"), "400" ("element")) -> (w306:string[])
                      n133 = property on="Instr3 Voltage (V)" class="Ring (strict)"(error in=w313, "Strings []"=w306) -> (error out=w312:errorcluster)  [unwired: 1 in, 1 out]
                    }
                    frame 8 {
                      n134 = Build Array("175" ("element"), "350" ("element")) -> (w329:string[])
                      n135 = property on="Instr1 Voltage (V)" class="Ring (strict)"(error in=w328, "Strings []"=w329) -> (error out=w327:errorcluster)  [unwired: 1 in, 1 out]
                      n136 = Build Array("0" ("element"), "0" ("element")) -> (w322:string[])
                      n137 = property on="Instr2 Voltage (V)" class="Ring (strict)"(error in=w327, "Strings []"=w322) -> (error out=w326:errorcluster)  [unwired: 1 in, 1 out]
                      n138 = Build Array("200" ("element"), "400" ("element")) -> (w319:string[])
                      n139 = property on="Instr3 Voltage (V)" class="Ring (strict)"(error in=w326, "Strings []"=w319) -> (error out=w325:errorcluster)  [unwired: 1 in, 1 out]
                    }
                    frame 1 {
                      n140 = Build Array("175" ("element"), "350" ("element")) -> (w339:string[])
                      n141 = property on="Instr1 Voltage (V)" class="Ring (strict)"(error in=w338, "Strings []"=w339) -> (error out=w337:errorcluster)  [unwired: 1 in, 1 out]
                      n142 = Build Array("0" ("element"), "0" ("element")) -> (w332:string[])
                      n143 = property on="Instr2 Voltage (V)" class="Ring (strict)"(error in=w337, "Strings []"=w332) -> (error out=w336:errorcluster)  [unwired: 1 in, 1 out]
                      n144 = property on="Instr3 Voltage (V)" class="Ring (strict)"(error in=w336, "Strings []"=w332) -> (error out=w335:errorcluster)  [unwired: 1 in, 1 out]
                    }
                    frame 14 {
                      n145 = Build Array("200" ("element"), "400" ("element")) -> (w349:string[])
                      n146 = property on="Instr1 Voltage (V)" class="Ring (strict)"(error in=w348, "Strings []"=w349) -> (error out=w347:errorcluster)  [unwired: 1 in, 1 out]
                      n147 = Build Array("175" ("element"), "350" ("element")) -> (w342:string[])
                      n148 = property on="Instr2 Voltage (V)" class="Ring (strict)"(error in=w347, "Strings []"=w342) -> (error out=w346:errorcluster)  [unwired: 1 in, 1 out]
                      n149 = property on="Instr3 Voltage (V)" class="Ring (strict)"(error in=w346, "Strings []"=w342) -> (error out=w345:errorcluster)  [unwired: 1 in, 1 out]
                    }
                    frame 2 {
                      n150 = Build Array("200" ("element"), "400" ("element")) -> (w359:string[])
                      n151 = property on="Instr1 Voltage (V)" class="Ring (strict)"(error in=w358, "Strings []"=w359) -> (error out=w357:errorcluster)  [unwired: 1 in, 1 out]
                      n152 = Build Array("0" ("element"), "0" ("element")) -> (w352:string[])
                      n153 = property on="Instr2 Voltage (V)" class="Ring (strict)"(error in=w357, "Strings []"=w352) -> (error out=w356:errorcluster)  [unwired: 1 in, 1 out]
                      n154 = property on="Instr3 Voltage (V)" class="Ring (strict)"(error in=w356, "Strings []"=w352) -> (error out=w355:errorcluster)  [unwired: 1 in, 1 out]
                    }
                    frame 3 {
                      n155 = Build Array("175" ("element"), "350" ("element")) -> (w362:string[])
                      n156 = property on="Instr1 Voltage (V)" class="Ring (strict)"(error in=w366, "Strings []"=w362) -> (error out=w365:errorcluster)  [unwired: 1 in, 1 out]
                      n157 = property on="Instr2 Voltage (V)" class="Ring (strict)"(error in=w365, "Strings []"=w362) -> (error out=w364:errorcluster)  [unwired: 1 in, 1 out]
                      n158 = property on="Instr3 Voltage (V)" class="Ring (strict)"(error in=w364, "Strings []"=w362) -> (error out=w363:errorcluster)  [unwired: 1 in, 1 out]
                    }
                    frame 9 {
                      n159 = Build Array("175" ("element"), "350" ("element")) -> (w372:string[])
                      n160 = property on="Instr1 Voltage (V)" class="Ring (strict)"(error in=w376, "Strings []"=w372) -> (error out=w375:errorcluster)  [unwired: 1 in, 1 out]
                      n161 = property on="Instr2 Voltage (V)" class="Ring (strict)"(error in=w375, "Strings []"=w372) -> (error out=w374:errorcluster)  [unwired: 1 in, 1 out]
                      n162 = Build Array("200" ("element"), "400" ("element")) -> (w369:string[])
                      n163 = property on="Instr3 Voltage (V)" class="Ring (strict)"(error in=w374, "Strings []"=w369) -> (error out=w373:errorcluster)  [unwired: 1 in, 1 out]
                    }
                    frame 4 {
                      n164 = Build Array("200" ("element"), "400" ("element")) -> (w379:string[])
                      n165 = property on="Instr1 Voltage (V)" class="Ring (strict)"(error in=w383, "Strings []"=w379) -> (error out=w382:errorcluster)  [unwired: 1 in, 1 out]
                      n166 = property on="Instr2 Voltage (V)" class="Ring (strict)"(error in=w382, "Strings []"=w379) -> (error out=w381:errorcluster)  [unwired: 1 in, 1 out]
                      n167 = property on="Instr3 Voltage (V)" class="Ring (strict)"(error in=w381, "Strings []"=w379) -> (error out=w380:errorcluster)  [unwired: 1 in, 1 out]
                    }
                  }
                }
              }
            }
          }
          event "btnSave": Value Change {
            (unwired) path "C:/Users/ico/Documents/Projects/UserFiles/Plugins/AcPwr/NHRGridSim/NHRRGS.ini" ("Accessors:PluginIniFilePath")
            w390 = TRUE ("StartMeas")
            # "Save the changes made to the configuration properties"
            n168 = event-data() -> ()  [unwired: 1 in, 1 out]
            n169 = disable-structure shown="Enabled" {
              disable-tunnel: [w413 w421] -> w389
              disable-tunnel: [w411 w422] -> w388
              disable-tunnel: w387 -> [w397 w422]
              disable-tunnel: w386 -> [w394 w421]
              frame Disabled {
                n170 = local read "Measurement RefreshTime (ms)"() -> (w393:u32)
                n171 = local read "Measurements"() -> (w395:T9)
                n172 = local read item#-1() -> (w396)
                n173 = To Variant(anything=w396) -> (Variant=w401:variant)
                n174 = To Variant(anything=w395) -> (Variant=w400:variant)
                n175 = call "WriteToBaseConfigVariant.vi"("Measurement RefreshTime (ms)"=w393, "error in (no error)"=w394, "Meas"=w400, "Config"=w401, "NHRGridSim in"=w397) -> ("error out"=w398:errorcluster, "NHRGridSim out"=w399:refnum<class "NHRGridSim.lvclass">)  [unwired: 5 in]
                n176 = Unbundle By Name(w396) -> ("Hardware"=w414)
                n177 = property class="NHRGridSim.lvclass"(reference=w399, error in=w398) -> (reference out=w411:refnum<class "NHRGridSim.lvclass">, error out=w408:errorcluster, "Accessors:PluginIniFilePath"=w392:path, "Accessors:BaseConfig"=w407:T15, "Accessors:BaseMeasurements"=w404:T17)
                n178 = disable-structure shown="Enabled" {
                  disable-tunnel: [w419 w420] -> w415
                  disable-tunnel: w414 -> [w418 w420]
                  frame Disabled {
                    n179 = Bundle By Name(cluster=w418, "Connected"=FALSE) -> (w419:cluster{})
                  }
                  frame Enabled {
                  }
                }
                n180 = Bundle By Name(cluster=w396, "Hardware"=w415) -> (w403:cluster{})
                n181 = To Variant(anything=w403) -> (Variant=w412:variant)
                n182 = To Variant(anything=w395) -> (Variant=w402:variant)
                n183 = call "WriteToBaseConfigVariant.vi"("Measurement RefreshTime (ms)"=w393, "error in (no error)"=w408, "Meas"=w402, "Config"=w412, "NHRGridSim in"=w411) -> ("error out"=w409:errorcluster, "NHRGridSim out"=w410:refnum<class "NHRGridSim.lvclass">)  [unwired: 5 in]
                n184 = call <vilib>:"Open Config Data.vi"("error in (no error)"=w409, "create file if necessary (T)"=FALSE, "configuration file path"=w392) -> ("error out"=w405:errorcluster, "refnum"=w406:T19)  [unwired: 6 in, 1 out]
                n185 = call-dynamic "WriteFile.vi"("RefreshTime"=w393, "Refnum in"=w406, "error in (no error)"=w405, "BaseMeasurements"=w404, "BaseConfiguration"=w407, "NHRGridSim in"=w410) -> ("error out"=w413:errorcluster)  [unwired: 4 in, 1 out]
              }
              frame Enabled {
              }
            }
          }
          event "btnSaveAs": Value Change {
            # "Save the configuration properties to a different file in the same location as the original file."
            n186 = event-data() -> ()  [unwired: 1 in, 1 out]
            n187 = disable-structure shown="Enabled" {
              disable-tunnel: [TRUE _] -> w427
              disable-tunnel: w426 -> [w457 w474]
              disable-tunnel: w425 -> [w456 w473]
              disable-tunnel: [w443 w473] -> w424
              disable-tunnel: [w441 w474] -> w423
              frame Disabled {
                w458 = "Type" ("section (optional)")
                n188 = local read "Measurement RefreshTime (ms)"() -> (w428:u32)
                n189 = property class="NHRGridSim.lvclass"(reference=w457, error in=w456) -> (reference out=w433:refnum<class "NHRGridSim.lvclass">, error out=w455:errorcluster, "Accessors:PluginIniFilePath"=w454:path)
                n190 = local read "Measurements"() -> (w430:T9)
                n191 = local read item#-1() -> (w431)
                n192 = Unbundle By Name(w431) -> ("Hardware"=w451)
                n193 = call "Prompt User for Input"("error in (no error)"=w455) -> ("File Name"=w453:string, "PluginType"=w459:string, "error out"=w460:errorcluster)  [unwired: 15 in, 1 out]
                n194 = Strip Path(path=w454) -> (stripped path=w465:path)  [unwired: 1 out]
                n195 = call "CheckFileName.vi"("Error In"=w460, "File Name in"=w453) -> ("Error Out"=w461:errorcluster, "File Name out"=w462:string)  [unwired: 8 in]
                n196 = disable-structure shown="Enabled" {
                  disable-tunnel: [w471 w472] -> w452
                  disable-tunnel: w451 -> [w470 w472]
                  frame Disabled {
                    n197 = Bundle By Name(cluster=w470, "Connected"=FALSE) -> (w471:cluster{})
                  }
                  frame Enabled {
                  }
                }
                n198 = Build Path(base path=w465, name or relative path=w462) -> (appended path=w464:path)
                n199 = Copy(8:w461, 10:w464, 11:w454) -> (0:w436:errorcluster, 3:w447:path)  [unwired: 2 in, 1 out]
                n200 = To Variant(anything=w430) -> (Variant=w429:variant)
                n201 = To Variant(anything=w431) -> (Variant=w432:variant)
                n202 = call "WriteToBaseConfigVariant.vi"("Measurement RefreshTime (ms)"=w428, "error in (no error)"=w436, "Meas"=w429, "Config"=w432, "NHRGridSim in"=w433) -> ("error out"=w435:errorcluster, "NHRGridSim out"=w434:refnum<class "NHRGridSim.lvclass">)  [unwired: 5 in]
                n203 = Bundle By Name(cluster=w431, "Hardware"=w452) -> (w450:cluster{})
                n204 = property class="NHRGridSim.lvclass"(reference=w434, error in=w435, "Accessors:PluginIniFilePath"=w447) -> (reference out=w441:refnum<class "NHRGridSim.lvclass">, error out=w442:errorcluster, "Accessors:PluginIniFilePath"=w446:path, "Accessors:BaseConfig"=w445:T15, "Accessors:BaseMeasurements"=w438:T17)
                n205 = To Variant(anything=w430) -> (Variant=w437:variant)
                n206 = To Variant(anything=w450) -> (Variant=w449:variant)
                n207 = call "WriteToBaseConfigVariant.vi"("Measurement RefreshTime (ms)"=w428, "error in (no error)"=w442, "Meas"=w437, "Config"=w449, "NHRGridSim in"=w441) -> ("error out"=w440:errorcluster, "NHRGridSim out"=w448:refnum<class "NHRGridSim.lvclass">)  [unwired: 5 in]
                n208 = call <vilib>:"Open Config Data.vi"("error in (no error)"=w440, "create file if necessary (T)"=TRUE, "configuration file path"=w446) -> ("error out"=w467:errorcluster, "refnum"=w466:T19)  [unwired: 6 in, 1 out]
                n209 = call <userlib>:"Write Key (Variant)__ogtk.vi"("section"=w458, "error in (no error)"=w467, "key-value"=w459, "key (optional)"=w458, "refnum"=w466) -> ("error out"=w439:errorcluster, "refnum out"=w444:T19)  [unwired: 5 in]
                n210 = call-dynamic "WriteFile.vi"("RefreshTime"=w428, "Refnum in"=w444, "error in (no error)"=w439, "BaseMeasurements"=w438, "BaseConfiguration"=w445, "NHRGridSim in"=w448) -> ("error out"=w443:errorcluster)  [unwired: 4 in, 1 out]
              }
              frame Enabled {
              }
            }
          }
        }
        n211 = Or(x=w18, y=w19) -> (x .or. y?=w20:bool)
      }
      "Changed" <- w17
      "Save As" <- w11
      n212 = property class="VI"(error in=w9, "FP.Behavior"=T11."Default" ("Front Panel Window:Behavior")) -> (error out=w15:errorcluster)  [unwired: 1 in, 1 out]
      n213 = property class="VI"(error in=w15, "FP.State"=T12."Standard" ("Front Panel Window:State")) -> (error out=w10:errorcluster)  [unwired: 1 in, 1 out]
    }
    frame Error {
    }
  }
  "MyPluginsBase out" <- w3
  "error out" <- w2
  n214 = disable-structure shown="Enabled" {
    frame Disabled {
      n215 = case shown="13" {
        selector: _ -> [_ _ _ _ _ _ _ _ _ _ _ _ _]
        tunnel: [w478 w481 w486 w491 w496 w501 w506 w511 w516 w520 w524 w528 w532] -> _
        tunnel: [1 1 3 3 3 3 3 3 3 2 2 2 2] -> _
        frame 0, 1, Default {
          n216 = Build Array("AC1") -> (w478:string[])
        }
        frame 2 {
          n217 = Build Array("DC1") -> (w481:string[])
        }
        frame 3 {
          n218 = Build Array("AC1", "AC2", "AC3") -> (w486:string[])
        }
        frame 4 {
          n219 = Build Array("DC1", "DC2", "DC3") -> (w491:string[])
        }
        frame 9 {
          n220 = Build Array("AC1", "AC2", "DC3") -> (w496:string[])
        }
        frame 10 {
          n221 = Build Array("AC1", "DC2", "DC3") -> (w501:string[])
        }
        frame 13 {
          n222 = Build Array("AC1", "DC2", "AC3") -> (w506:string[])
        }
        frame 14 {
          n223 = Build Array("DC1", "AC2", "AC3") -> (w511:string[])
        }
        frame 15 {
          n224 = Build Array("DC1", "AC2", "DC3") -> (w516:string[])
        }
        frame 5, 7 {
          n225 = Build Array("AC1", "AC3") -> (w520:string[])
        }
        frame 6, 8 {
          n226 = Build Array("AC1", "DC3") -> (w524:string[])
        }
        frame 11 {
          n227 = Build Array("DC1", "AC3") -> (w528:string[])
        }
        frame 12 {
          n228 = Build Array("DC1", "DC3") -> (w532:string[])
        }
      }
    }
    frame Enabled {
    }
  }
